vi "Derivative (2D).vi"(8 "error in (no error)":errorcluster, 10 "Axis Array":dbl[](array[numeric]), 11 "Conductance":dbl[][](graph)) -> (0 "error out":errorcluster, 3 "Transconductance":dbl[][](graph))   [LabVIEW 2016, in "Retrieve and Visualize.lvclass"]
uses:
  Retrieve and Visualize.lvclass
  <userlib>/LevyLab/XY Utilities/subVIs/Append (double array).vi
  <userlib>/LevyLab/XY Utilities/subVIs/Derivative (single).vi
  <userlib>/LevyLab/XY Utilities/xy_utilities.lvlib
panel:
  in  "Type":enum16{"dy/dx vs x", "dx/dy vs y"}(ring)
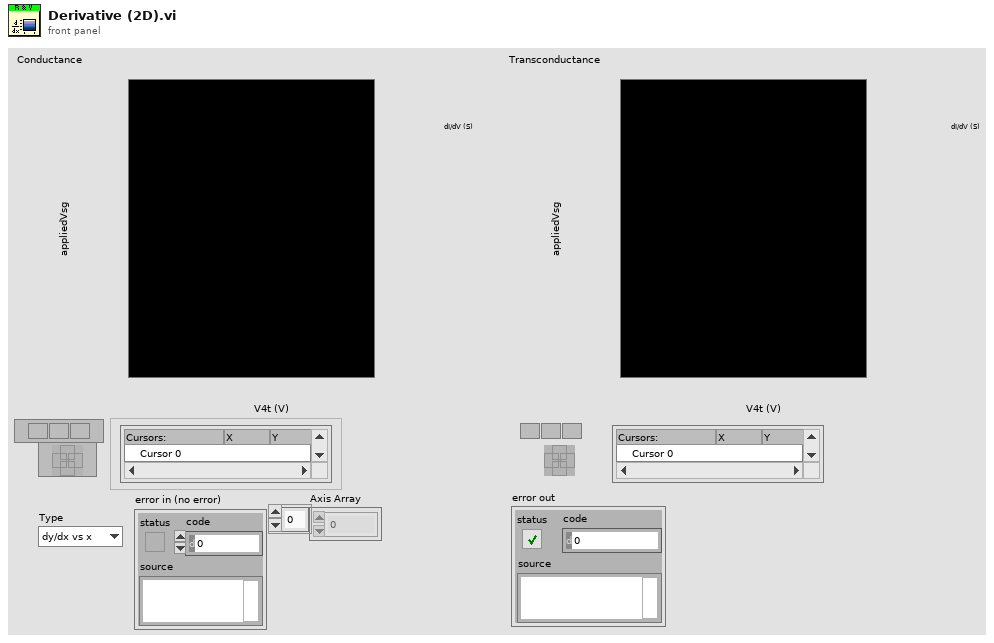
[diagram p1: front panel]
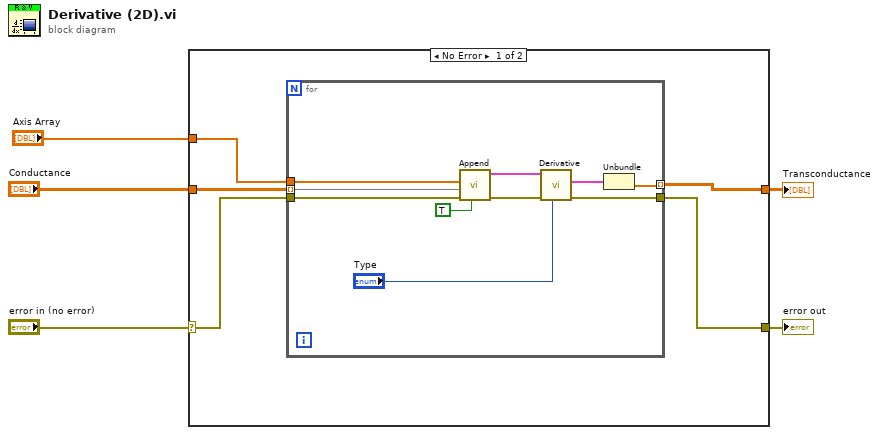
[diagram p0: block diagram]
diagram:
  n1 = case shown="No Error" "error in (no error)" {
    selector: "error in (no error)" -> [w7 w22]
    tunnel: "Axis Array" -> [w10 _]
    tunnel: "Conductance" -> [w9 w21]
    tunnel: [w8 w21] -> w3
    tunnel: [w6 w22] -> w2
    frame No Error {
      n2 = for {
        tunnel: w9 -> [w17] mode=indexing
        tunnel: w10 -> [w18]
        tunnel: [w19] -> w8 mode=indexing
        tunnel: [w13] -> w6
        tunnel: w7 -> [w12]
        n3 = call-poly <userlib>:"Append.vi"("Reset"=TRUE, "error in (no error)"=w12, "Y-array"=w17, "X-array"=w18) -> ("error out"=w14:errorcluster, "XY-data out"=w16:cluster{"X-array":dbl[], "Y-array":dbl[]})  [unwired: 6 in]
        n4 = call-poly <userlib>:"Derivative.vi"("Type"="Type", "error in (no error)"=w14, "XY-data"=w16) -> ("error out"=w13:errorcluster, "Differential out"=w20:cluster{"X-array":dbl[], "Y-array":dbl[]})  [unwired: 6 in, 1 out]
        n5 = Unbundle(w20) -> ("Y-array"=w19:dbl[])  [unwired: 1 out]
      }
    }
    frame Error {
    }
  }
  "Transconductance" <- w3
  "error out" <- w2
